vi "log analysis_gps.vi"() -> ()   [LabVIEW 2018] (continued)
02000000,d426,15824;SOL_COMPUTED,NARROW_FLOAT,-1.000000000,128.837829590,37.580234528,0.0,360.000000000,180.000000000,\"631T\",23,8,8,7,04,00,20,33*aad36c56\n\tsystem status\tnormal 2 28.100000 0 0\trobot status\t162.287043\t121.769386\t7.931900\t-0.515576\t0.455981\t-8.309532\t0.300000\t0.043000\n\t\n15:15:16.1\tlog_raw\tgps_raw\t#DUALANTENNAHEADINGA,USB3,0,46.5,FINESTEERING,2107,281734.100,02000000,d426,15824;SOL_COMPUTED,L1_FLOAT,-1.000000000,224.733520508,68.118484497,0.0,40.168888092,35.261268616,\"631T\",23,9,9,8,04,00,20,32*6f92941a\n\tsystem status\tnormal 2 28.000000 0 0\trobot status\t162.425752\t121.748646\t7.934200\t-0.505297\t0.498713\t-7.822119\t0.330000\t-0.013000\n\t\n15:15:16.6\tlog_raw\tgps_raw\t#DUALANTENNAHEADINGA,USB3,0,49.0,FINESTEERING,2107,281734.600,02000000,d426,15824;SOL_COMPUTED,L1_FLOAT,-1.000000000,224.765914917,68.098785400,0.0,40.323402405,35.416801453,\"631T\",24,9,9,8,04,00,20,32*7247d44b\n\tsystem status\tnormal 2 28.000000 0 0\trobot status\t162.566104\t121.728918\t7.937400\t-0.642162\t0.281643\t-7.263950\t0.334000\t-0.022000\n\t\n15:15:17.1\tlog_raw\tgps_raw\t#DUALANTENNAHEADINGA,USB3,0,49.0,FINESTEERING,2107,281735.100,02000000,d426,15824;SOL_COMPUTED,NARROW_FLOAT,-1.000000000,130.053359985,14.075355530,0.0,360.000000000,180.000000000,\"631T\",24,8,8,7,04,00,20,33*3c5b7a30\n\tsystem status\tnormal 2 28.000000 0 0\trobot status\t162.703780\t121.710709\t7.940600\t-0.736035\t0.242485\t-6.590546\t0.270000\t0.061000\n\t\n15:15:17.6\tlog_raw\tgps_raw\t#DUALANTENNAHEADINGA,USB3,0,49.5,FINESTEERING,2107,281735.600,02000000,d426,15824;SOL_COMPUTED,NARROW_FLOAT,-1.000000000,129.132507324,11.961747169,0.0,360.000000000,180.000000000,\"631T\",23,8,8,7,04,00,20,33*3d51ce5b\n\tsystem status\tnormal 2 28.000000 0 0\trobot status\t162.840537\t121.687841\t7.943400\t-0.790275\t0.331459\t-6.069682\t0.236000\t0.113000\n\t\n15:15:18.1\tlog_raw\tgps_raw\t#DUALANTENNAHEADINGA,USB3,0,49.0,FINESTEERING,2107,281736.100,02000000,d426,15824;SOL_COMPUTED,NARROW_FLOAT,-1.000000000,66.459640503,-9.324951172,0.0,167.365310669,180.000000000,\"631T\",23,11,11,7,04,00,20,33*cd3bb081\n\tsystem status\tnormal 2 28.000000 0 0\trobot status\t162.977193\t121.667344\t7.944900\t-0.701534\t0.221863\t-5.523543\t0.376000\t-0.103000\n\t\n15:15:18.6\tlog_raw\tgps_raw\t#DUALANTENNAHEADINGA,USB3,0,49.0,FINESTEERING,2107,281736.600,02000000,d426,15824;SOL_COMPUTED,NARROW_FLOAT,-1.000000000,65.953575134,-8.853302002,0.0,164.536880493,180.000000000,\"631T\",23,11,11,7,04,00,20,33*7a71c18e\n\tsystem status\tnormal 2 28.000000 0 0\trobot status\t163.118877\t121.649897\t7.948900\t-0.553992\t0.083987\t-5.065243\t0.332000\t-0.028000\n\t\n15:15:19.1\tlog_raw\tgps_raw\t#DUALANTENNAHEADINGA,USB3,0,48.0,FINESTEERING,2107,281737.100,02000000,d426,15824;SOL_COMPUTED,NARROW_FLOAT,-1.000000000,177.908920288,86.914611816,0.0,360.000000000,93.604774475,\"631T\",23,9,9,9,04,00,20,32*986b758d\n\tsystem status\tnormal 2 28.000000 0 0\trobot status\t163.259043\t121.634913\t7.953300\t-0.493468\t0.027328\t-4.685907\t0.370000\t-0.104000\n\t\n15:15:19.6\tlog_raw\tgps_raw\t#DUALANTENNAHEADINGA,USB3,0,48.0,FINESTEERING,2107,281737.600,02000000,d426,15824;SOL_COMPUTED,NARROW_FLOAT,-1.000000000,175.774688721,87.167266846,0.0,360.000000000,89.855789185,\"631T\",24,8,8,8,04,00,20,32*9d4057da\n\tsystem status\tnormal 2 28.100000 0 0\trobot status\t163.400214\t121.619860\t7.957900\t-0.604019\t-0.174535\t-4.390079\t0.270000\t0.058000\n\t\n15:15:20.1\tlog_raw\tgps_raw\t#DUALANTENNAHEADINGA,USB3,0,48.0,FINESTEERING,2107,281738.100,02000000,d426,15824;SOL_COMPUTED,NARROW_FLOAT,-1.000000000,69.591072083,21.682659149,0.0,219.854476929,180.000000000,\"631T\",24,11,11,8,04,00,20,33*690f967f\n\tsystem status\tnormal 2 28.100000 0 0\trobot status\t163.541877\t121.605719\t7.962200\t-0.638008\t-0.259636\t-4.163410\t0.238000\t0.086000\n\t\n15:15:20.6\tlog_raw\tgps_raw\t\tsystem status\tnormal 2 28.100000 0 0\trobot status\t163.684912\t121.588071\t7.966500\t-0.574519\t-0.050612\t-4.063875\t0.336000\t-0.052000\n\t\n15:15:21.1\tlog_raw\tgps_raw\t#DUALANTENNAHEADINGA,USB3,0,44.0,FINESTEERING,2107,281739.100,02000000,d426,15824;SOL_COMPUTED,NARROW_FLOAT,-1.000000000,64.034339905,-17.544586182,0.0,156.327194214,180.000000000,\"631T\",24,11,11,10,04,00,20,23*2589d380\n\tsystem status\tnormal 2 28.100000 0 0\trobot status\t163.825678\t121.571157\t7.970500\t-0.474647\t0.048927\t-4.119423\t0.280000\t0.031000\n\t\n15:15:21.6\tlog_raw\tgps_raw\t\tsystem status\tnormal 2 28.200000 0 0\trobot status\t163.967418\t121.552468\t7.973500\t-0.433512\t0.045180\t-4.183395\t0.279000\t0.023000\n\t\n15:15:22.1\tlog_raw\tgps_raw\t#DUALANTENNAHEADINGA,USB3,0,44.0,FINESTEERING,2107,281740.100,02000000,d426,15824;SOL_COMPUTED,NARROW_FLOAT,-1.000000000,74.082733154,-10.455871582,0.0,242.974914551,180.000000000,\"631T\",25,10,10,8,04,00,20,33*2f825e02\n\tsystem status\tnormal 2 28.200000 0 0\trobot status\t164.107869\t121.533673\t7.976000\t-0.484376\t0.023753\t-4.275160\t0.292000\t0.001000\n\t\n15:15:22.6\tlog_raw\tgps_raw\t\tsystem status\tnormal 2 28.200000 0 0\trobot status\t164.246429\t121.506929\t7.974700\t-0.479451\t0.055607\t-4.352606\t0.298000\t0.002000\n\t\n15:15:23.1\tlog_raw\tgps_raw\t#DUALANTENNAHEADINGA,USB3,0,47.0,FINESTEERING,2107,281741.100,02000000,d426,15824;SOL_COMPUTED,NARROW_FLOAT,-1.000000000,85.015144348,31.514696121,0.0,312.612518311,180.000000000,\"631T\",25,11,11,10,04,00,20,33*b44ad5e5\n\tsystem status\tnormal 2 28.200000 0 0\trobot status\t164.384072\t121.480395\t7.973700\t-0.358400\t0.052205\t-4.435176\t0.296000\t-0.004000\n\t\n15:15:23.6\tlog_raw\tgps_raw\t#DUALANTENNAHEADINGA,USB3,0,47.0,FINESTEERING,2107,281741.600,02000000,d426,15824;SOL_COMPUTED,NARROW_FLOAT,-1.000000000,83.672279358,32.063629150,0.0,308.060882568,180.000000000,\"631T\",26,11,11,9,04,00,20,33*4b707776\n\tsystem status\tnormal 2 28.200000 0 0\trobot status\t164.530836\t121.453220\t7.971100\t-0.159969\t-0.070035\t-4.573891\t0.300000\t-0.008000\n\t\n15:15:24.1\tlog_raw\tgps_raw\t\tsystem status\tnormal 2 28.200000 0 0\trobot status\t164.671620\t121.428851\t7.968700\t-0.225099\t-0.038968\t-4.709220\t0.146000\t0.017000\n\t\n15:15:24.6\tlog_raw\tgps_raw\t#DUALANTENNAHEADINGA,USB3,0,48.0,FINESTEERING,2107,281742.600,02000000,d426,15824;SOL_COMPUTED,NARROW_FLOAT,-1.000000000,70.145378113,-51.275817871,0.0,227.918136597,180.000000000,\"631T\",25,9,9,9,04,00,20,33*d9969f72\n\tsystem status\tnormal 2 28.200000 0 0\trobot status\t164.681911\t121.417195\t7.969000\t-0.139098\t-0.127113\t-4.691425\t-0.003000\t-0.005000\n\t\n15:15:25.1\tlog_raw\tgps_raw\t\tsystem status\tnormal 2 28.200000 0 0\trobot status\t164.682503\t121.407898\t7.969700\t-0.165244\t-0.111582\t-4.696632\t0.000000\t0.000000\n\t\n15:15:25.6\tlog_raw\tgps_raw\t#DUALANTENNAHEADINGA,USB3,0,44.0,FINESTEERING,2107,281743.600,02000000,d426,15824;SOL_COMPUTED,NARROW_FLOAT,-1.000000000,80.124595642,-25.270904541,0.0,308.231628418,180.000000000,\"631T\",24,11,11,8,04,00,20,33*e319a4f8\n\tsystem status\tnormal 2 28.200000 0 0\trobot status\t164.681523\t121.398031\t7.970300\t-0.161453\t-0.099720\t-4.699516\t0.000000\t0.000000\n\t\n15:15:26.1\tlog_raw\tgps_raw\t#DUALANTENNAHEADINGA,USB3,0,44.0,FINESTEERING,2107,281744.100,02000000,d426,15824;SOL_COMPUTED,NARROW_FLOAT,-1.000000000,88.668289185,-42.090301514,0.0,218.729476929,180.000000000,\"631T\",27,12,12,8,04,00,20,33*7e036603\n\tsystem status\tnormal 2 28.200000 0 0\trobot status\t164.682496\t121.388269\t7.970500\t-0.157645\t-0.102462\t-4.701254\t0.000000\t0.000000\n\t\n15:15:26.6\tlog_raw\tgps_raw\t\tsystem status\tnormal 2 28.200000 0 0\trobot status\t164.682998\t121.381077\t7.969800\t-0.155032\t-0.099826\t-4.698427\t0.000000\t0.000000\n\t\n15:15:27.1\tlog_raw\tgps_raw\t#DUALANTENNAHEADINGA,USB3,0,43.0,FINESTEERING,2107,281745.100,02000000,d426,15824;SOL_COMPUTED,L1_FLOAT,-1.000000000,76.229156494,-52.514221191,0.0,343.746551514,180.000000000,\"631T\",24,8,8,8,04,00,20,22*58ffa7a9\n\tsystem status\tnormal 2 28.200000 0 0\trobot status\t164.683786\t121.374068\t7.969500\t-0.153230\t-0.100561\t-4.694181\t0.000000\t0.000000\n\t\n15:15:27.6\tlog_raw\tgps_raw\t#INSPVAXA,USB3,0,43.0,FINESTEERING,2107,281745.650,02000000,471d,15824;INS_ALIGNMENT_COMPLETE,INS_RTKFIXED,37.37122376712,126.72269430723,7.9696,22.3000,0.0009,-0.0216,0.0069,-0.151476991,-0.103231506,94.688643057,0.4242,0.2996,0.5710,0.1152,0.0935,0.0773,0.1637,0.1653,5.0964,0f000001,0*7621de5b\n\tsystem status\tnormal 2 28.200000 0 0\trobot status\t164.685080\t121.367878\t7.969600\t-0.151477\t-0.103232\t-4.688643\t0.000000\t0.000000\n\t\n15:15:28.1\tlog_raw\tgps_raw\t#DUALANTENNAHEADINGA,USB3,0,43.0,FINESTEERING,2107,281746.100,02000000,d426,15824;SOL_COMPUTED,NARROW_FLOAT,-1.000000000,80.487289429,-0.437042236,0.0,264.792785645,180.000000000,\"631T\",23,11,11,9,04,00,20,33*333581cd\n\tsystem status\tnormal 2 28.200000 0 0\trobot status\t164.685546\t121.363224\t7.969900\t-0.150285\t-0.104238\t-4.680634\t0.000000\t0.000000\n\t\n15:15:28.6\tlog_raw\tgps_raw\t#INSPVAXA,USB3,0,48.5,FINESTEERING,2107,281746.650,02000000,471d,15824;INS_ALIGNMENT_COMPLETE,INS_RTKFIXED,37.37122367686,126.72269432693,7.9700,22.3000,-0.0006,-0.0203,0.0085,-0.151258490,-0.103499239,94.673524903,0.4235,0.2995,0.5674,0.1146,0.0934,0.0772,0.1636,0.1652,5.0926,0f000001,0*5a88747a\n\tsystem status\tnormal 2 28.200000 0 0\trobot status\t164.686825\t121.357860\t7.970000\t-0.151258\t-0.103499\t-4.673525\t0.000000\t0.000000\n\t\n15:15:29.1\tlog_raw\tgps_raw\t#DUALANTENNAHEADINGA,USB3,0,47.0,FINESTEERING,2107,281747.100,02000000,d426,15824;SOL_COMPUTED,NARROW_FLOAT,-1.000000000,79.948493958,-1.148895264,0.0,261.968414307,180.000000000,\"631T\",25,11,11,8,04,00,20,33*bccd161e\n\tsystem status\tnormal 2 28.200000 0 0\trobot status\t164.687444\t121.353759\t7.970800\t-0.150960\t-0.103722\t-4.666938\t0.000000\t0.000000\n\t\n15:15:29.6\tlog_raw\tgps_raw\t#INSPVAXA,USB3,0,47.0,FINESTEERING,2107,281747.650,02000000,471d,15824;INS_ALIGNMENT_COMPLETE,INS_RTKFIXED,37.37122361083,126.72269434828,7.9719,22.3000,-0.0025,-0.0192,0.0107,-0.148677227,-0.104675299,94.662876541,0.4231,0.2994,0.5645,0.1138,0.0934,0.0773,0.1636,0.1650,5.0876,0f000001,0*63e2391f\n\tsystem status\tnormal 2 28.200000 0 0\trobot status\t164.688716\t121.350532\t7.971900\t-0.148677\t-0.104675\t-4.662877\t0.000000\t0.000000\n\t\n15:15:30.1\tlog_raw\tgps_raw\t#DUALANTENNAHEADINGA,USB3,0,47.0,FINESTEERING,2107,281748.100,02000000,d426,15824;SOL_COMPUTED,NARROW_FLOAT,-1.000000000,79.773033142,-38.986785889,0.0,161.515747070,180.000000000,\"631T\",26,14,14,9,04,00,20,23*3f0231ce\n\tsystem status\tnormal 2 28.200000 0 0\trobot status\t164.689395\t121.347700\t7.973400\t-0.147638\t-0.104974\t-4.659202\t0.000000\t0.000000\n\t\n15:15:30.6\tlog_raw\tgps_raw\t#INSPVAXA,USB3,0,47.0,FINESTEERING,2107,281748.650,02000000,471d,15824;INS_ALIGNMENT_COMPLETE,INS_RTKFIXED,37.37122355418,126.72269437706,7.9761,22.3000,-0.0041,-0.0183,0.0125,-0.147280099,-0.105053583,94.655580641,0.4227,0.2992,0.5623,0.1131,0.0933,0.0773,0.1635,0.1648,5.0828,0f000001,0*cff9a17d\n\tsystem status\tnormal 2 28.200000 0 0\trobot status\t164.691265\t121.344244\t7.976100\t-0.147280\t-0.105054\t-4.655581\t0.000000\t0.000000\n\t\n15:15:31.1\tlog_raw\tgps_raw\t#DUALANTENNAHEADINGA,USB3,0,47.0,FINESTEERING,2107,281749.100,02000000,d426,15824;SOL_COMPUTED,NARROW_FLOAT,-1.000000000,78.765502930,-35.557800293,0.0,142.700469971,180.000000000,\"631T\",25,9,9,9,04,00,20,23*972183bf\n\tsystem status\tnormal 2 28.100000 0 0\trobot status\t164.703454\t121.340433\t7.979200\t-0.126703\t0.027217\t-4.432636\t0.218000\t-0.001000\n\t\n15:15:31.6\tlog_raw\tgps_raw\t#INSPVAXA,USB3,0,47.0,FINESTEERING,2107,281749.650,02000000,471d,15824;INS_ALIGNMENT_COMPLETE,INS_RTKFIXED,37.37122336848,126.72269668314,7.9846,22.3000,-0.0207,0.2294,0.0088,-0.275967163,-0.168126378,94.547495368,0.4219,0.2990,0.5605,0.1123,0.0932,0.0774,0.1635,0.1647,5.0793,0f000001,0*31f4ca89\n\tsystem status\tnormal 2 28.200000 0 0\trobot status\t164.895534\t121.323631\t7.984600\t-0.275967\t-0.168126\t-4.547495\t0.249000\t0.098000\n\t\n15:15:32.1\tlog_raw\tgps_raw\t#DUALANTENNAHEADINGA,USB3,0,47.0,FINESTEERING,2107,281750.100,02000000,d426,15824;SOL_COMPUTED,NARROW_FLOAT,-1.000000000,73.333755493,-58.579284668,0.0,229.934936523,180.000000000,\"631T\",23,9,9,9,04,00,20,23*088e0644\n\tsystem status\tnormal 2 28.100000 0 0\trobot status\t165.015435\t121.310202\t7.988900\t-0.193033\t-0.068842\t-4.487636\t0.286000\t0.107000\n\t\n15:15:32.6\tlog_raw\tgps_raw\t#INSPVAXA,USB3,0,49.0,FINESTEERING,2107,281750.650,02000000,471d,15824;INS_ALIGNMENT_COMPLETE,INS_RTKFIXED,37.37122306940,126.72269984285,7.9912,22.3000,-0.0257,0.2957,0.0077,-0.057724950,-0.163350878,94.045578333,0.4218,0.2990,0.5600,0.1154,0.0932,0.0775,0.1634,0.1646,5.0783,0f000001,0*27ab5aaa\n\tsystem status\tnormal 2 28.100000 0 0\trobot status\t165.175416\t121.290432\t7.991200\t-0.057725\t-0.163351\t-4.045578\t0.226000\t0.166000\n\t\n15:15:33.1\tlog_raw\tgps_raw\t#INSPVAXA,USB3,0,44.0,FINESTEERING,2107,281751.150,02000000,471d,15824;INS_ALIGNMENT_COMPLETE,INS_RTKFIXED,37.37122292112,126.72270145835,7.9931,22.3000,-0.0258,0.2880,0.0101,-0.111536572,-0.252430525,93.709532324,0.4176,0.2990,0.5591,0.1145,0.0931,0.0775,0.1634,0.1645,5.0797,0f000001,0*615311ce\n\tsystem status\tnormal 2 28.100000 0 0\trobot status\t165.318514\t121.273972\t7.993100\t-0.111537\t-0.252431\t-3.709532\t0.247000\t0.096000\n\t\n15:15:33.6\tlog_raw\tgps_raw\t#DUALANTENNAHEADINGA,USB3,0,44.0,FINESTEERING,2107,281751.600,02000000,d426,15824;SOL_COMPUTED,NARROW_FLOAT,-1.000000000,110.156936646,-9.428588867,0.0,360.000000000,180.000000000,\"631T\",23,8,8,8,04,00,20,33*43819e80\n\tsystem status\tnormal 2 28.000000 0 0\trobot status\t165.448114\t121.260717\t7.996600\t-0.244048\t-0.440131\t-3.218956\t0.367000\t-0.071000\n\t\n15:15:34.1\tlog_raw\tgps_raw\t#INSPVAXA,USB3,0,48.0,FINESTEERING,2107,281752.150,02000000,471d,15824;INS_ALIGNMENT_COMPLETE,INS_RTKFIXED,37.37122265407,126.72270470547,8.0012,22.3000,-0.0341,0.2842,0.0130,-0.222146581,-0.505161594,92.535665637,0.4393,0.3011,0.5700,0.1180,0.0937,0.0785,0.1633,0.1649,5.0792,0f000001,0*a665f62f\n\tsystem status\tnormal 2 28.000000 0 0\trobot status\t165.606139\t121.244328\t8.001200\t-0.222147\t-0.505162\t-2.535666\t0.243000\t0.112000\n\t\n15:15:34.6\tlog_raw\tgps_raw\t\tsystem status\tnormal 2 28.000000 0 0\trobot status\t165.737807\t121.231977\t8.005700\t-0.196982\t-0.562881\t-2.053303\t0.295000\t0.031000\n\t\n15:15:35.1\tlog_raw\tgps_raw\t#INSPVAXA,USB3,0,47.0,FINESTEERING,2107,281753.150,02000000,471d,15824;INS_ALIGNMENT_COMPLETE,INS_RTKFIXED,37.37122240940,126.72270799161,8.0105,22.3000,-0.0212,0.2738,0.0106,-0.057702421,-0.540115409,91.679699760,0.4576,0.3026,0.5817,0.1199,0.0939,0.0793,0.1633,0.1651,5.0754,0f000001,0*cdf942d8\n\tsystem status\tnormal 2 28.000000 0 0\trobot status\t165.897220\t121.217168\t8.010500\t-0.057702\t-0.540115\t-1.679700\t0.344000\t-0.053000\n\t\n15:15:35.6\tlog_raw\tgps_raw\t\tsystem status\tnormal 2 28.100000 0 0\trobot status\t166.025860\t121.206663\t8.013100\t-0.153728\t-0.418900\t-1.370203\t0.269000\t0.059000\n\t\n15:15:36.1\tlog_raw\tgps_raw\t#INSPVAXA,USB3,0,49.5,FINESTEERING,2107,281754.150,02000000,471d,15824;INS_ALIGNMENT_COMPLETE,INS_RTKFIXED,37.37122220677,126.72271122628,8.0166,22.3000,-0.0162,0.2741,0.0138,-0.137895898,-0.319145604,91.130640627,0.4709,0.3035,0.5925,0.1202,0.0941,0.0798,0.1633,0.1651,5.0690,0f000001,0*5011df6e\n\tsystem status\tnormal 2 28.100000 0 0\trobot status\t166.183742\t121.194673\t8.016600\t-0.137896\t-0.319146\t-1.130641\t0.245000\t0.081000\n\t\n15:15:36.6\tlog_raw\tgps_raw\t\tsystem status\tnormal 2 28.100000 0 0\trobot status\t166.313373\t121.185926\t8.017600\t-0.339771\t-0.390316\t-1.051788\t0.237000\t0.079000\n\t\n15:15:37.1\tlog_raw\tgps_raw\t#INSPVAXA,USB3,0,47.5,FINESTEERING,2107,281755.150,02000000,471d,15824;INS_ALIGNMENT_COMPLETE,INS_RTKFIXED,37.37122201064,126.72271448049,8.0208,22.3000,-0.0166,0.2736,0.0165,-0.348957996,-0.224906485,91.007651183,0.4789,0.3039,0.6014,0.1198,0.0941,0.0802,0.1633,0.1650,5.0614,0f000001,0*7ee29d08\n\tsystem status\tnormal 2 28.100000 0 0\trobot status\t166.471994\t121.172900\t8.020800\t-0.348958\t-0.224906\t-1.007651\t0.390000\t-0.153000\n\t\n15:15:37.6\tlog_raw\tgps_raw\t#INSPVAXA,USB3,0,47.5,FINESTEERING,2107,281755.650,02000000,471d,15824;INS_ALIGNMENT_COMPLETE,INS_RTKFIXED,37.37122187648,126.72271611793,8.0227,22.3000,-0.0203,0.2843,0.0276,-0.262004326,-0.178495771,91.033181464,0.4789,0.3039,0.6014,0.1198,0.0941,0.0802,0.1633,0.1650,5.0614,0f000001,0*fdcbd20c\n\tsystem status\tnormal 2 28.200000 0 0\trobot status\t166.617036\t121.158007\t8.022700\t-0.262004\t-0.178496\t-1.033181\t0.308000\t-0.013000\n\t\n15:15:38.1\tlog_raw\tgps_raw\t#INSPVAXA,USB3,0,48.5,FINESTEERING,2107,281756.150,02000000,471d,15824;INS_ALIGNMENT_COMPLETE,INS_RTKFIXED,37.37122173906,126.72271771096,8.0239,22.3000,-0.0196,0.2676,0.0157,-0.262264917,-0.227266763,91.141814343,0.4824,0.3038,0.6077,0.1190,0.0941,0.0803,0.1632,0.1648,5.0544,0f000001,0*6ba67688\n\tsystem status\tnormal 2 28.200000 0 0\trobot status\t166.758144\t121.142753\t8.023900\t-0.262265\t-0.227267\t-1.141814\t0.291000\t-0.002000\n\t\n15:15:38.6\tlog_raw\tgps_raw\t#INSPVAXA,USB3,0,48.5,FINESTEERING,2107,281756.650,02000000,471d,15824;INS_ALIGNMENT_COMPLETE,INS_RTKFIXED,37.37122160314,126.72271932823,8.0233,22.3000,-0.0269,0.2666,0.0159,-0.432031669,-0.241379053,91.270317292,0.4824,0.3038,0.6077,0.1190,0.0941,0.0803,0.1632,0.1648,5.0544,0f000001,0*d136edd6\n\tsystem status\tnormal 2 28.200000 0 0\trobot status\t166.901399\t121.127665\t8.023300\t-0.432032\t-0.241379\t-1.270317\t0.294000\t-0.007000\n\t\n15:15:39.1\tlog_raw\tgps_raw\t#INSPVAXA,USB3,0,46.0,FINESTEERING,2107,281757.150,02000000,471d,15824;INS_ALIGNMENT_COMPLETE,INS_RTKFIXED,37.37122146617,126.72272086261,8.0239,22.3000,-0.0238,0.2505,0.0126,-0.539342745,-0.282143344,91.361763043,0.4827,0.3037,0.6118,0.1183,0.0941,0.0803,0.1632,0.1647,5.0490,0f000001,0*c068de04\n\tsystem status\tnormal 2 28.200000 0 0\trobot status\t167.037312\t121.112461\t8.023900\t-0.539343\t-0.282143\t-1.361763\t0.211000\t-0.053000\n\t\n15:15:39.6\tlog_raw\tgps_raw\t\tsystem status\tnormal 2 28.200000 0 0\trobot status\t167.041973\t121.102348\t8.023100\t-0.585274\t-0.285310\t-1.348305\t-0.008000\t-0.012000\n\t\n15:15:40.1\tlog_raw\tgps_raw\t#INSPVAXA,USB3,0,45.0,FINESTEERING,2107,281758.150,02008000,471d,15824;INS_ALIGNMENT_COMPLETE,INS_RTKFIXED,37.37122126174,126.72272085859,8.0222,22.3000,-0.0253,0.0078,0.0138,-0.584106594,-0.271120528,91.359411557,0.4805,0.3034,0.6136,0.1183,0.0941,0.0802,0.1631,0.1646,5.0450,0f000001,0*5d21a2ee\n\tsystem status\tnormal 2 28.200000 0 0\trobot status\t167.036956\t121.089772\t8.022200\t-0.584107\t-0.271121\t-1.359412\t0.000000\t0.000000\n\t\n15:15:40.6\tlog_raw\tgps_raw\t\tsystem status\tnormal 2 28.200000 0 0\trobot status\t167.034826\t121.080403\t8.020600\t-0.576169\t-0.273378\t-1.355877\t0.000000\t0.000000\n\t\n15:15:41.1\tlog_raw\tgps_raw\t#INSPVAXA,USB3,0,48.0,FINESTEERING,2107,281759.150,02008000,471d,15824;INS_ALIGNMENT_COMPLETE,INS_RTKFIXED,37.37122108214,126.72272080985,8.0198,22.3000,-0.0260,-0.0094,0.0141,-0.568558330,-0.274735846,91.351120657,0.4775,0.3029,0.6135,0.1183,0.0941,0.0800,0.1631,0.1645,5.0455,0f000001,0*eb7ab8d8\n\tsystem status\tnormal 2 28.200000 0 0\trobot status\t167.032639\t121.069840\t8.019800\t-0.568558\t-0.274736\t-1.351121\t0.000000\t0.000000\n\t\n15:15:41.6\tlog_raw\tgps_raw\t#INSPVAXA,USB3,0,48.0,FINESTEERING,2107,281759.650,02008000,471d,15824;INS_ALIGNMENT_COMPLETE,INS_RTKFIXED,37.37122103098,126.72272079622,8.0204,22.3000,-0.0250,-0.0120,0.0146,-0.568680900,-0.276246354,91.350467693,0.4775,0.3029,0.6135,0.1183,0.0941,0.0800,0.1631,0.1645,5.0455,0f000001,0*f26d72a9\n\tsystem status\tnormal 2 28.200000 0 0\trobot status\t167.031431\t121.064162\t8.020400\t-0.568681\t-0.276246\t-1.350468\t0.000000\t0.000000\n\t\n15:15:42.1\tlog_raw\tgps_raw\t\tsystem status\tnormal 2 28.200000 0 0\trobot status\t167.029589\t121.059632\t8.021200\t-0.570148\t-0.276311\t-1.348928\t0.000000\t0.000000\n\t\n15:15:42.6\tlog_raw\tgps_raw\t#INSPVAXA,USB3,0,49.0,FINESTEERING,2107,281760.650,02008000,471d,15824;INS_ALIGNMENT_COMPLETE,INS_RTKFIXED,37.37122097057,126.72272075488,8.0199,22.3000,-0.0212,-0.0129,0.0148,-0.569283262,-0.275679751,91.347037233,0.5005,0.3048,0.6288,0.1214,0.0945,0.0808,0.1631,0.1649,5.0468,0f000001,0*fe34bbca\n\tsystem status\tnormal 2 28.200000 0 0\trobot status\t167.027769\t121.057457\t8.019900\t-0.569283\t-0.275680\t-1.347037\t0.000000\t0.000000\n\t\n15:15:43.1\tlog_raw\tgps_raw\t#INSPVAXA,USB3,0,45.0,FINESTEERING,2107,281761.150,02008000,471d,15824;INS_ALIGNMENT_COMPLETE,INS_RTKFIXED,37.37122095791,126.72272073406,8.0193,22.3000,-0.0189,-0.0135,0.0143,-0.568902262,-0.276160283,91.348963154,0.5200,0.3063,0.6436,0.1235,0.0947,0.0816,0.1630,0.1651,5.0472,0f000001,0*0a850e4d\n\tsystem status\tnormal 2 28.200000 0 0\trobot status\t167.025925\t121.056052\t8.019300\t-0.568902\t-0.276160\t-1.348963\t0.000000\t0.000000\n\t\n15:15:43.6\tlog_raw\tgps_raw\t#INSPVAXA,USB3,0,45.0,FINESTEERING,2107,281761.650,02008000,471d,15824;INS_ALIGNMENT_COMPLETE,INS_RTKFIXED,37.37122095627,126.72272072968,8.0191,22.3000,-0.0178,0.0000,0.0152,-0.570572969,-0.261989481,91.327306860,0.5200,0.3063,0.6436,0.1235,0.0947,0.0816,0.1630,0.1651,5.0472,0f000001,0*036a1cc5\n\tsystem status\tnormal 2 28.200000 0 0\trobot status\t167.025537\t121.055870\t8.019100\t-0.570573\t-0.261989\t-1.327307\t0.033000\t-0.004000\n\t\n15:15:44.1\tlog_raw\tgps_raw\t#INSPVAXA,USB3,0,48.5,FINESTEERING,2107,281762.150,02008000,471d,15824;INS_ALIGNMENT_COMPLETE,INS_RTKFIXED,37.37122093950,126.72272215279,8.0206,22.3000,-0.0488,0.3741,0.0233,-0.705475481,-0.265236590,91.294421038,0.5354,0.3074,0.6573,0.1254,0.0948,0.0822,0.1629,0.1651,5.0466,0f000001,0*f62868a6\n\tsystem status\tnormal 2 28.100000 0 0\trobot status\t167.151594\t121.054006\t8.020600\t-0.705475\t-0.265237\t-1.294421\t0.336000\t0.059000\n\t\n15:15:44.6\tlog_raw\tgps_raw\t#INSPVAXA,USB3,0,48.5,FINESTEERING,2107,281762.650,02008000,471d,15824;INS_ALIGNMENT_COMPLETE,INS_RTKFIXED,37.37122090398,126.72272383903,8.0212,22.3000,-0.0171,0.2083,0.0195,-0.539847805,-0.389561252,91.382608507,0.5354,0.3074,0.6573,0.1254,0.0948,0.0822,0.1629,0.1651,5.0466,0f000001,0*ee4bab04\n\tsystem status\tnormal 2 28.200000 0 0\trobot status\t167.300958\t121.050061\t8.021200\t-0.539848\t-0.389561\t-1.382609\t0.282000\t0.032000\n\t\n15:15:45.1\tlog_raw\tgps_raw\t#INSPVAXA,USB3,0,45.5,FINESTEERING,2107,281763.150,02000000,471d,15824;INS_ALIGNMENT_COMPLETE,INS_RTKFIXED,37.37122088109,126.72272535886,8.0227,22.3000,-0.0346,0.3404,0.0283,-0.600883432,-0.278437530,91.419884915,0.5438,0.3081,0.6694,0.1254,0.0948,0.0826,0.1629,0.1651,5.0479,0f000001,0*0f3b6f6b\n\tsystem status\tnormal 2 28.100000 0 0\trobot status\t167.435582\t121.047518\t8.022700\t-0.600883\t-0.278438\t-1.419885\t0.317000\t0.027000\n\t\n15:15:45.6\tlog_raw\tgps_raw\t#INSPVAXA,USB3,0,45.5,FINESTEERING,2107,281763.650,02000000,471d,15824;INS_ALIGNMENT_COMPLETE,INS_RTKFIXED,37.37122084767,126.72272697455,8.0246,22.3000,-0.0147,0.2375,0.0201,-0.753001308,-0.365484631,91.444706948,0.5438,0.3081,0.6694,0.1254,0.0948,0.0826,0.1629,0.1651,5.0479,0f000001,0*dfc03d63\n\tsystem status\tnormal 2 28.200000 0 0\trobot status\t167.578698\t121.043806\t8.024600\t-0.753001\t-0.365485\t-1.444707\t0.278000\t-0.010000\n\t\n15:15:46.1\tlog_raw\tgps_raw\t#INSPVAXA,USB3,0,48.5,FINESTEERING,2107,281764.150,02000000,471d,15824;INS_ALIGNMENT_COMPLETE,INS_RTKFIXED,37.37122080817,126.72272865797,8.0273,22.3000,-0.0183,0.2610,0.0199,-0.883754251,-0.497263643,91.594297223,0.5508,0.3085,0.6797,0.1258,0.0948,0.0829,0.1629,0.1651,5.0491,0f000001,0*98c9c36a\n\tsystem status\tnormal 2 28.200000 0 0\trobot status\t167.727812\t121.039419\t8.027300\t-0.883754\t-0.497264\t-1.594297\t0.289000\t0.012000\n\t\n15:15:46.6\tlog_raw\tgps_raw\t#INSPVAXA,USB3,0,48.5,FINESTEERING,2107,281764.650,02000000,471d,15824;INS_ALIGNMENT_COMPLETE,INS_RTKFIXED,37.37122075325,126.72273024996,8.0307,22.3000,-0.0230,0.2873,0.0155,-0.910536369,-0.571169391,91.698573448,0.5508,0.3085,0.6797,0.1258,0.0948,0.0829,0.1629,0.1651,5.0491,0f000001,0*a48c0ed7\n\tsystem status\tnormal 2 28.200000 0 0\trobot status\t167.868828\t121.033321\t8.030700\t-0.910536\t-0.571169\t-1.698573\t0.308000\t0.000000\n\t\n15:15:47.1\tlog_raw\tgps_raw\t#INSPVAXA,USB3,0,49.5,FINESTEERING,2107,281765.150,02000000,471d,15824;INS_ALIGNMENT_COMPLETE,INS_RTKFIXED,37.37122068841,126.72273183543,8.0343,22.3000,-0.0165,0.2820,0.0133,-0.835088790,-0.555071717,91.791979713,0.5558,0.3086,0.6882,0.1257,0.0948,0.0832,0.1628,0.1650,5.0496,0f000001,0*cba52910\n\tsystem status\tnormal 2 28.200000 0 0\trobot status\t168.009266\t121.026122\t8.034300\t-0.835089\t-0.555072\t-1.791980\t0.302000\t-0.005000\n\t\n15:15:47.6\tlog_raw\tgps_raw\t#INSPVAXA,USB3,0,49.5,FINESTEERING,2107,281765.650,02000000,471d,15824;INS_ALIGNMENT_COMPLETE,INS_RTKFIXED,37.37122061486,126.72273346284,8.0365,22.3000,-0.0171,0.2746,0.0152,-0.832834423,-0.571575823,91.924169920,0.5558,0.3086,0.6882,0.1257,0.0948,0.0832,0.1628,0.1650,5.0496,0f000001,0*526b2e24\n\tsystem status\tnormal 2 28.200000 0 0\trobot status\t168.153420\t121.017956\t8.036500\t-0.832834\t-0.571576\t-1.924170\t0.299000\t-0.009000\n\t\n15:15:48.1\tlog_raw\tgps_raw\t#INSPVAXA,USB3,0,49.0,FINESTEERING,2107,281766.150,02000000,471d,15824;INS_ALIGNMENT_COMPLETE,INS_RTKFIXED,37.37122054097,126.72273507488,8.0385,22.3000,-0.0218,0.2706,0.0128,-1.000637631,-0.672076774,92.055365430,0.5592,0.3087,0.6949,0.1259,0.0948,0.0833,0.1628,0.1650,5.0498,0f000001,0*57bf3361\n\tsystem status\tnormal 2 28.200000 0 0\trobot status\t168.296212\t121.009753\t8.038500\t-1.000638\t-0.672077\t-2.055365\t0.299000\t-0.010000\n\t\n15:15:48.6\tlog_raw\tgps_raw\t#INSPVAXA,USB3,0,49.0,FINESTEERING,2107,281766.650,02000000,471d,15824;INS_ALIGNMENT_COMPLETE,INS_RTKFIXED,37.37122044479,126.72273670968,8.0412,22.3000,-0.0285,0.2846,0.0116,-1.092573740,-0.740242490,92.171373793,0.5592,0.3087,0.6949,0.1259,0.0948,0.0833,0.1628,0.1650,5.0498,0f000001,0*1c223ea9\n\tsystem status\tnormal 2 28.200000 0 0\trobot status\t168.441019\t120.999075\t8.041200\t-1.092574\t-0.740242\t-2.171374\t0.303000\t-0.010000\n\t\n15:15:49.1\tlog_raw\tgps_raw\t#INSPVAXA,USB3,0,48.0,FINESTEERING,2107,281767.150,02000000,471d,15824;INS_ALIGNMENT_COMPLETE,INS_RTKFIXED,37.37122033445,126.72273829026,8.0449,22.3000,-0.0305,0.2613,0.0217,-0.977094539,-0.639903649,92.271203612,0.5614,0.3086,0.7003,0.1258,0.0947,0.0834,0.1628,0.1649,5.0495,0f000001,0*5c3b8fb1\n\tsystem status\tnormal 2 28.200000 0 0\trobot status\t168.581025\t120.986826\t8.044900\t-0.977095\t-0.639904\t-2.271204\t0.295000\t-0.023000\n\t\n15:15:49.6\tlog_raw\tgps_raw\t#INSPVAXA,USB3,0,48.0,FINESTEERING,2107,281767.650,02000000,471d,15824;INS_ALIGNMENT_COMPLETE,INS_RTKFIXED,37.37122021827,126.72273994335,8.0476,22.3000,-0.0288,0.2733,0.0197,-0.964628632,-0.656119186,92.463441538,0.5614,0.3086,0.7003,0.1258,0.0947,0.0834,0.1628,0.1649,5.0495,0f000001,0*cc7927eb\n\tsystem status\tnormal 2 28.200000 0 0\trobot status\t168.727453\t120.973929\t8.047600\t-0.964629\t-0.656119\t-2.463442\t0.298000\t-0.013000\n\t\n15:15:50.1\tlog_raw\tgps_raw\t#INSPVAXA,USB3,0,48.0,FINESTEERING,2107,281768.150,02000000,471d,15824;INS_ALIGNMENT_COMPLETE,INS_RTKFIXED,37.37122009872,126.72274157958,8.0500,22.3000,-0.0294,0.2847,0.0191,-0.946431620,-0.566462229,92.660906936,0.5627,0.3085,0.7043,0.1259,0.0947,0.0835,0.1628,0.1649,5.0496,0f000001,0*cc13fb9d\n\tsystem status\tnormal 2 28.200000 0 0\trobot status\t168.872387\t120.960658\t8.050000\t-0.946432\t-0.566462\t-2.660907\t0.300000\t-0.019000\n\t\n15:15:50.6\tlog_raw\tgps_raw\t#INSPVAXA,USB3,0,49.0,FINESTEERING,2107,281768.650,02000000,471d,15824;INS_ALIGNMENT_COMPLETE,INS_RTKFIXED,37.37121997801,126.72274320142,8.0509,22.3000,-0.0214,0.2856,0.0260,-1.015543433,-0.231279609,92.847402266,0.5627,0.3085,0.7043,0.1259,0.0947,0.0835,0.1628,0.1649,5.0496,0f000001,0*22053697\n\tsystem status\tnormal 2 28.200000 0 0\trobot status\t169.016047\t120.947258\t8.050900\t-1.015543\t-0.231280\t-2.847402\t0.300000\t-0.018000\n\t\n15:15:51.1\tlog_raw\tgps_raw\t\tsystem status\tnormal 2 28.200000 0 0\trobot status\t169.161838\t120.931907\t8.052500\t-0.947911\t0.033902\t-3.024219\t0.302000\t-0.009000\n\t\n15:15:51.6\tlog_raw\tgps_raw\t#INSPVAXA,USB3,0,46.5,FINESTEERING,2107,281769.650,02000000,471d,15824;INS_ALIGNMENT_COMPLETE,INS_RTKFIXED,37.37121967893,126.72274645196,8.0567,22.3000,-0.0370,0.2793,0.0333,-0.818626182,0.216920532,93.214992796,0.5635,0.3085,0.7075,0.1258,0.0947,0.0835,0.1628,0.1649,5.0499,0f000001,0*792e5a9d\n\tsystem status\tnormal 2 28.200000 0 0\trobot status\t169.303975\t120.914059\t8.056700\t-0.818626\t0.216921\t-3.214993\t0.301000\t-0.017000\n\t\n15:15:52.1\tlog_raw\tgps_raw\t\tsystem status\tnormal 2 28.200000 0 0\trobot status\t169.448482\t120.896336\t8.060800\t-0.845783\t0.315070\t-3.412635\t0.297000\t-0.009000\n\t\n15:15:52.6\tlog_raw\tgps_raw\t\tsystem status\tnormal 2 28.200000 0 0\trobot status\t169.592546\t120.876946\t8.063800\t-0.838684\t0.237497\t-3.632390\t0.302000\t-0.011000\n\t\n15:15:53.1\tlog_raw\tgps_raw\t#INSPVAXA,USB3,0,48.5,FINESTEERING,2107,281771.150,02000000,471d,15824;INS_ALIGNMENT_COMPLETE,INS_RTKFIXED,37.37121916335,126.72275134411,8.0669,22.3000,-0.0460,0.2833,0.0183,-0.792418480,0.032350312,93.864070762,0.5648,0.3085,0.7116,0.1262,0.0947,0.0836,0.1628,0.1649,5.0523,0f000001,0*03020e62\n\tsystem status\tnormal 2 28.200000 0 0\trobot status\t169.737313\t120.856829\t8.066900\t-0.792418\t0.032350\t-3.864071\t0.296000\t-0.007000\n\t\n15:15:53.6\tlog_raw\tgps_raw\t\tsystem status\tnormal 2 28.200000 0 0\trobot status\t169.880959\t120.836597\t8.069700\t-0.704803\t-0.086987\t-4.075804\t0.297000\t-0.006000\n\t\n15:15:54.1\tlog_raw\tgps_raw\t#INSPVAXA,USB3,0,47.0,FINESTEERING,2107,281772.150,02000000,471d,15824;INS_ALIGNMENT_COMPLETE,INS_RTKFIXED,37.37121879734,126.72275457125,8.0729,22.3000,-0.0562,0.2927,0.0149,-0.701118394,-0.215535385,94.262257179,0.5652,0.3086,0.7131,0.1264,0.0948,0.0837,0.1628,0.1649,5.0539,0f000001,0*6742cf9b\n\tsystem status\tnormal 2 28.200000 0 0\trobot status\t170.023168\t120.816202\t8.072900\t-0.701118\t-0.215535\t-4.262257\t0.299000\t0.001000\n\t\n15:15:54.6\tlog_raw\tgps_raw\t\tsystem status\tnormal 2 28.200000 0 0\trobot status\t170.164461\t120.795574\t8.075000\t-0.726816\t-0.261675\t-4.437290\t0.300000\t0.006000\n\t\n15:15:55.1\tlog_raw\tgps_raw\t#INSPVAXA,USB3,0,47.5,FINESTEERING,2107,281773.150,02000000,471d,15824;INS_ALIGNMENT_COMPLETE,INS_RTKFIXED,37.37121842061,126.72275777876,8.0764,22.3000,-0.0402,0.2880,0.0117,-0.782099339,-0.380092330,94.588227053,0.5655,0.3117,0.7220,0.1266,0.0954,0.0843,0.1628,0.1649,5.0554,0f000001,0*2c781ada\n\tsystem status\tnormal 2 28.200000 0 0\trobot status\t170.307284\t120.774385\t8.076400\t-0.782099\t-0.380092\t-4.588227\t0.297000\t0.005000\n\t\n15:15:55.6\tlog_raw\tgps_raw\t\tsystem status\tnormal 2 28.200000 0 0\trobot status\t170.447622\t120.752993\t8.077900\t-0.844276\t-0.626810\t-4.709261\t0.298000\t0.009000\n\t\n15:15:56.1\tlog_raw\tgps_raw\t\tsystem status\tnormal 2 28.200000 0 0\trobot status\t170.591761\t120.730533\t8.080600\t-0.766459\t-0.768182\t-4.771713\t0.284000\t0.000000\n\t\n15:15:56.6\tlog_raw\tgps_raw\t#INSPVAXA,USB3,0,47.5,FINESTEERING,2107,281774.650,02000000,471d,15824;INS_ALIGNMENT_COMPLETE,INS_RTKFIXED,37.37121790104,126.72276172821,8.0844,22.3000,-0.0056,-0.1159,0.0265,-0.829469010,-1.054819962,94.805665616,0.5657,0.3125,0.7262,0.1269,0.0954,0.0845,0.1628,0.1649,5.0568,0f000001,0*5083390f\n\tsystem status\tnormal 2 28.200000 0 0\trobot status\t170.657120\t120.716713\t8.084400\t-0.829469\t-1.054820\t-4.805666\t-0.048000\t0.000000\n\t\n15:15:57.1\tlog_raw\tgps_raw\t\tsystem status\tnormal 2 28.200000 0 0\trobot status\t170.634895\t120.710290\t8.088400\t-0.811869\t-1.011582\t-4.772675\t0.001000\t0.002000\n\t\n15:15:57.6\tlog_raw\tgps_raw\t#INSPVAXA,USB3,0,45.5,FINESTEERING,2107,281775.650,02000000,471d,15824;INS_ALIGNMENT_COMPLETE,INS_RTKFIXED,37.37121775993,126.72276174880,8.0908,22.3000,-0.0341,0.2302,0.0228,-0.820870768,-0.784541706,94.618919565,0.5657,0.3121,0.7276,0.1285,0.0952,0.0845,0.1627,0.1649,5.0580,0f000001,0*ef5961e6\n\tsystem status\tnormal 2 28.100000 0 0\trobot status\t170.658944\t120.701052\t8.090800\t-0.820871\t-0.784542\t-4.618920\t0.230000\t-0.016000\n\t\n15:15:58.1\tlog_raw\tgps_raw\t\tsystem status\tnormal 2 28.200000 0 0\trobot status\t170.807010\t120.681576\t8.092700\t-0.785705\t-1.480331\t-4.708494\t0.031000\t-0.005000\n\t\n15:15:58.6\tlog_raw\tgps_raw\t\tsystem status\tnormal 2 28.200000 0 0\trobot status\t170.763842\t120.681403\t8.093300\t-0.826722\t-0.935584\t-4.563170\t0.098000\t0.021000\n\t\n15:15:59.1\tlog_raw\tgps_raw\t#INSPVAXA,USB3,0,49.5,FINESTEERING,2107,281777.150,02000000,471d,15824;INS_ALIGNMENT_COMPLETE,INS_RTKFIXED,37.37121742515,126.72276471335,8.0933,22.3000,-0.0434,0.3635,0.0199,-0.788823341,-1.034155621,94.704274658,0.5667,0.3105,0.7263,0.1288,0.0950,0.0844,0.1627,0.1648,5.0605,0f000001,0*58cfd0fe\n\tsystem status\tnormal 2 28.200000 0 0\trobot status\t170.921539\t120.663891\t8.093300\t-0.788823\t-1.034156\t-4.704275\t0.372000\t-0.085000\n\t\n15:15:59.6\tlog_raw\tgps_raw\t\tsystem status\tnormal 2 28.100000 0 0\trobot status\t171.047476\t120.651764\t8.092900\t-0.833508\t-0.756016\t-4.545820\t0.299000\t0.009000\n\t\n15:16:00.1\tlog_raw\tgps_raw\t\tsystem status\tnormal 2 28.100000 0 0\trobot status\t171.190074\t120.635839\t8.090400\t-0.892806\t-0.490182\t-4.350230\t0.205000\t0.132000\n\t\n15:16:00.6\tlog_raw\tgps_raw\t\tsystem status\tnormal 2 28.100000 0 0\trobot status\t171.330385\t120.610836\t8.078300\t-0.869431\t-0.472348\t-3.990617\t0.241000\t0.100000\n\t\n15:16:01.1\tlog_raw\tgps_raw\t\tsystem status\tnormal 2 28.000000 0 0\trobot status\t171.469953\t120.589634\t8.069300\t-0.916855\t-0.487523\t-3.389294\t0.336000\t-0.037000\n\t\n15:16:01.6\tlog_raw\tgps_raw\t\tsystem status\tnormal 2 28.000000 0 0\trobot status\t171.614157\t120.573968\t8.068500\t-0.749279\t-0.534396\t-2.778435\t0.280000\t0.056000\n\t\n15:16:02.1\tlog_raw\tgps_raw\t\tsystem status\tnormal 2 27.900000 0 0\trobot status\t171.754741\t120.560806\t8.068100\t-0.729336\t-0.814607\t-2.083031\t0.311000\t0.015000\n\t\n15:16:02.6\tlog_raw\tgps_raw\t#INSPVAXA,USB3,0,49.5,FINESTEERING,2107,281780.650,02000000,471d,15824;INS_ALIGNMENT_COMPLETE,INS_RTKFIXED,37.37121639807,126.72277573033,8.0654,22.3000,-0.0075,0.2871,0.0244,-0.701767133,-0.824742936,91.476878975,0.4298,0.3000,0.6003,0.1163,0.0939,0.0789,0.1625,0.1636,5.0634,0f000001,0*3e81e8f3\n\tsystem status\tnormal 2 28.000000 0 0\trobot status\t171.897405\t120.549881\t8.065400\t-0.701767\t-0.824743\t-1.476879\t0.280000\t0.051000\n\t\n15:16:03.1\tlog_raw\tgps_raw\t\tsystem status\tnormal 2 28.000000 0 0\trobot status\t172.040165\t120.541002\t8.061400\t-0.888421\t-0.659852\t-0.839585\t0.203000\t0.152000\n\t\n15:16:03.6\tlog_raw\tgps_raw\t\tsystem status\tnormal 2 28.100000 0 0\trobot status\t172.183489\t120.531922\t8.055100\t-1.024816\t-0.805912\t-0.396205\t0.346000\t-0.050000\n\t\n15:16:04.1\tlog_raw\tgps_raw\t#INSPVAXA,USB3,0,49.0,FINESTEERING,2107,281782.150,02000000,471d,15824;INS_ALIGNMENT_COMPLETE,INS_RTKFIXED,37.37121614895,126.72278060077,8.0494,22.3000,-0.0125,0.2941,0.0170,-0.958151284,-0.907972358,90.050842278,0.4192,0.2995,0.5761,0.1162,0.0938,0.0788,0.1624,0.1635,5.0656,0f000001,0*79d70d48\n\tsystem status\tnormal 2 28.100000 0 0\trobot status\t172.328820\t120.522224\t8.049400\t-0.958151\t-0.907972\t-0.050842\t0.400000\t-0.127000\n\t\n15:16:04.6\tlog_raw\tgps_raw\t\tsystem status\tnormal 2 28.100000 0 0\trobot status\t172.474796\t120.513361\t8.045800\t-0.979784\t-1.055898\t0.181148\t0.405000\t-0.143000\n\t\n15:16:05.1\tlog_raw\tgps_raw\t\tsystem status\tnormal 2 28.100000 0 0\trobot status\t172.621853\t120.506373\t8.043000\t-1.205147\t-1.289641\t0.278849\t0.255000\t0.073000\n\t\n15:16:05.6\tlog_raw\tgps_raw\t\tsystem status\tnormal 2 28.200000 0 0\trobot status\t172.766127\t120.499985\t8.039800\t-1.308059\t-1.342637\t0.217677\t0.342000\t-0.065000\n\t\n15:16:06.1\tlog_raw\tgps_raw\t\tsystem status\tnormal 2 28.200000 0 0\trobot status\t172.910156\t120.492387\t8.036200\t-1.292665\t-1.198328\t0.177557\t0.305000\t-0.009000\n\t\n15:16:06.6\tlog_raw\tgps_raw\t\tsystem status\tnormal 2 28.200000 0 0\trobot status\t173.053484\t120.483209\t8.031700\t-1.105104\t-0.966771\t0.129149\t0.278000\t0.004000\n\t\n15:16:07.1\tlog_raw\tgps_raw\t\tsystem status\tnormal 2 28.200000 0 0\trobot status\t173.202194\t120.476498\t8.026000\t-1.439210\t-1.085585\t-0.040698\t0.298000\t-0.016000\n\t\n15:16:07.6\tlog_raw\tgps_raw\t\tsystem status\tnormal 2 28.200000 0 0\trobot status\t173.344261\t120.465452\t8.018400\t-1.534448\t-1.182356\t-0.149377\t0.294000\t-0.017000\n\t\n15:16:08.1\tlog_raw\tgps_raw\t\tsystem status\tnormal 2 28.200000 0 0\trobot status\t173.477391\t120.453069\t8.012300\t-1.509363\t-1.269202\t-0.176457\t0.186000\t0.043000\n\t\n15:16:08.6\tlog_raw\tgps_raw\t\tsystem status\tnormal 2 28.200000 0 0\trobot status\t173.456845\t120.440874\t8.009600\t-1.432366\t-1.213471\t-0.208652\t-0.013000\t-0.002000\n\t\n15:16:09.1\tlog_raw\tgps_raw\t\tsystem status\tnormal 2 28.200000 0 0\trobot status\t173.476956\t120.430661\t8.007300\t-1.479699\t-1.230610\t-0.253017\t0.008000\t-0.012000\n\t\n15:16:09.6\tlog_raw\tgps_raw\t\tsystem status\tnormal 2 28.200000 0 0\trobot status\t173.481553\t120.423546\t8.006500\t-1.473812\t-1.229416\t-0.248387\t0.000000\t0.000000\n\t\n15:16:10.1\tlog_raw\tgps_raw\t\tsystem status\tnormal 2 28.200000 0 0\trobot status\t173.487355\t120.417410\t8.005900\t-1.475440\t-1.230091\t-0.245287\t0.000000\t0.000000\n\t\n15:16:10.6\tlog_raw\tgps_raw\t\tsystem status\tnormal 2 28.200000 0 0\trobot status\t173.491255\t120.414135\t8.005100\t-1.475052\t-1.230691\t-0.238436\t0.000000\t0.000000\n\t\n15:16:11.1\tlog_raw\tgps_raw\t\tsystem status\tnormal 2 28.200000 0 0\trobot status\t173.494877\t120.410878\t8.004000\t-1.475644\t-1.230768\t-0.235402\t0.000000\t0.000000\n\t\n15:16:11.7\tlog_raw\tgps_raw\t\tsystem status\tnormal 2 28.200000 0 0\trobot status\t173.496911\t120.408413\t8.001000\t-1.477928\t-1.231203\t-0.234499\t0.000000\t0.000000\n\t\n15:16:12.2\tlog_raw\tgps_raw\t\tsystem status\tnormal 2 28.200000 0 0\trobot status\t173.498949\t120.406555\t7.998100\t-1.476876\t-1.231867\t-0.234212\t0.000000\t0.000000\n\t\n15:16:12.7\tlog_raw\tgps_raw\t\tsystem status\tnormal 2 28.200000 0 0\trobot status\t173.500318\t120.406193\t7.995100\t-1.477837\t-1.230381\t-0.235589\t0.000000\t0.000000\n\t\n15:16:13.2\tlog_raw\tgps_raw\t\tsystem status\tnormal 2 28.200000 0 0\trobot status\t173.501701\t120.406166\t7.992500\t-1.477810\t-1.228353\t-0.234764\t0.000000\t0.000000\n\t\n15:16:13.7\tlog_raw\tgps_raw\t\tsystem status\tnormal 2 28.200000 0 0\trobot status\t173.501519\t120.407176\t7.989800\t-1.476214\t-1.227329\t-0.235742\t0.000000\t0.000000\n\t\n15:16:14.2\tlog_raw\tgps_raw\t\tsystem status\tnormal 2 28.200000 0 0\trobot status\t173.498204\t120.411545\t7.982400\t-1.475964\t-1.227051\t-0.238850\t0.000000\t0.000000\n\t\n15:16:14.7\tlog_raw\tgps_raw\t\tsystem status\tnormal 2 28.200000 0 0\trobot status\t173.485668\t120.425323\t7.960000\t-1.476534\t-1.223732\t-0.254439\t0.000000\t0.000000\n\t\n15:16:15.2\tlog_raw\tgps_raw\t\tsystem status\tnormal 2 28.200000 0 0\trobot status\t173.476390\t120.435688\t7.942500\t-1.476120\t-1.221173\t-0.267555\t0.000000\t0.000000\n\t\n15:16:15.7\tlog_raw\tgps_raw\t\tsystem status\tnormal 2 28.200000 0 0\trobot status\t173.475101\t120.436395\t7.936900\t-1.475779\t-1.221176\t-0.267521\t0.000000\t0.000000\n\t\n15:16:16.2\tlog_raw\tgps_raw\t#INSPVAXA,USB3,0,48.0,FINESTEERING,2107,281794.200,02000000,471d,15824;INS_ALIGNMENT_COMPLETE,INS_RTKFIXED,37.37121538500,126.72279353221,7.9323,22.3000,0.0019,0.0033,0.0055,-1.472038191,-1.222257427,90.266116104,0.2743,0.1995,0.4008,0.0352,0.0349,0.0325,0.1516,0.1495,5.0388,0f000005,0*12f5b6da\n\tsystem status\tnormal 2 28.200000 
